vi "KE622x -- Delta Mode Get Params.vi"(0 "Resource In":refnum<visa-resource-name>, 1 "Check For SCPI Errors? (T)":bool=TRUE, 11 "error in (no error)":errorcluster) -> (4 "Resource Out (dupl)":refnum<visa-resource-name>, 8 "Delta Mode Params":T1={"High Level (A)"=0.001, "Low Level (A)"=-0.001, "Delay (s)"=0.002, "Num Cycles Mode"=enum."Finite Count", "Finite Count"=1, "Abort On\nCompliance?"=FALSE, "Cold Swithing\nMode Enabled?"=FALSE} {"Finite Count" min=1 max=65536; "Low Level (A)" min=-0.105 max=0.0 format="%.3p"; "High Level (A)" min=0.0 max=0.105 format="%.3p"; "Delay (s)" min=0.001 max=9999.999 format="%.3f"}, 15 "error out":errorcluster)   [LabVIEW 2020, in "Keithley 622x.lvlib"]
doc: "Returns the parameters for 'Delta' measurements. Note that performing this measurement implies that the 622x is being used in conjuction with a 2182/2182A nano-voltmeter."
uses:
  Keithley 622x.lvlib
  Typedefs/KE622x -- Delta Mode Params.ctl
  Low Level/Typedefs/KE622x -- Delta PDelta Mode High Level.ctl
  Low Level/Typedefs/KE622x -- Delta PDelta Mode Low Level.ctl
  Low Level/Typedefs/KE622x -- Delta DCon Mode Delay.ctl
  Low Level/Typedefs/KE622x -- Delta PDelta Mode Num Cycles Mode.ctl
  Low Level/Typedefs/KE622x -- Delta PDelta Mode Num Cycles.ctl
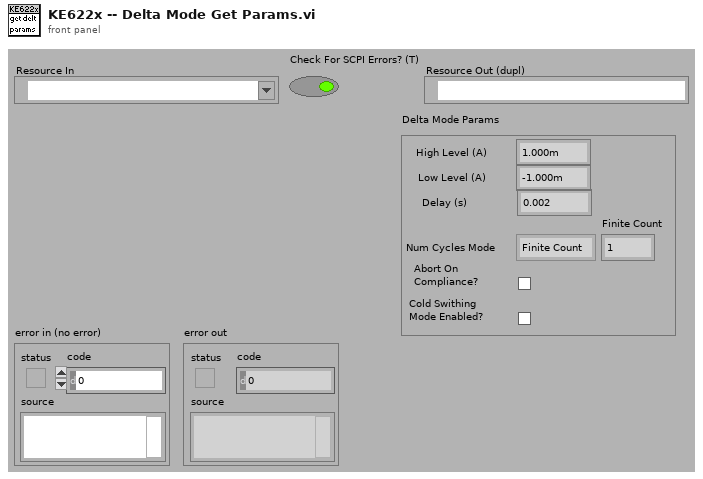
[diagram p1: front panel]
types:
  T1 = typedef "Keithley 622x.lvlib/KE622x -- Delta Mode Params.ctl" = cluster{"High Level (A)":T2, "Low Level (A)":T3, "Delay (s)":T4, "Num Cycles Mode":T5, "Finite Count":T6, "Abort On\nCompliance?":bool, "Cold Swithing\nMode Enabled?":bool}
  T2 = typedef "Keithley 622x.lvlib/KE622x -- Delta PDelta Mode High Level.ctl" = dbl
  T3 = typedef "Keithley 622x.lvlib/KE622x -- Delta PDelta Mode Low Level.ctl" = dbl
  T4 = typedef "Keithley 622x.lvlib/KE622x -- Delta DCon Mode Delay.ctl" = dbl
  T5 = typedef "Keithley 622x.lvlib/KE622x -- Delta PDelta Mode Num Cycles Mode.ctl" = enum16{"Finite Count", "Infinite"}
  T6 = typedef "Keithley 622x.lvlib/KE622x -- Delta PDelta Mode Num Cycles.ctl" = u32
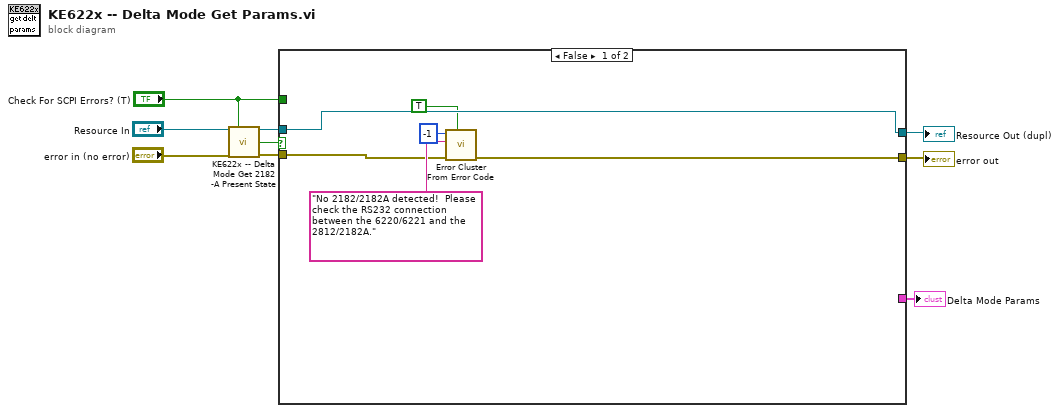
[diagram p0: block diagram]
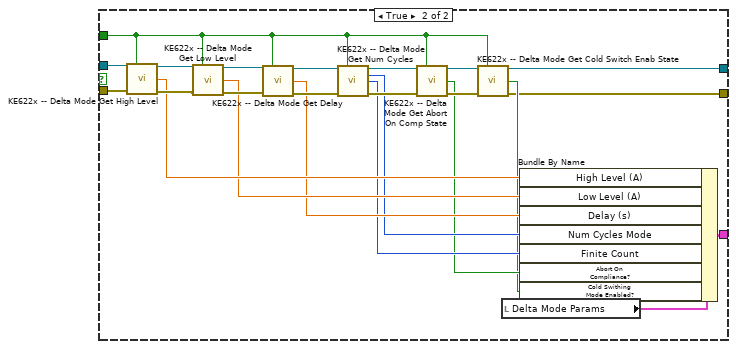
[diagram p2: hidden frame]
diagram:
  n1 = call "KE622x -- Delta Mode Get 2182 -A Present State.vi"("Resource In"="Resource In", "Check For SCPI Errors? (T)"="Check For SCPI Errors? (T)", "error in (no error)"="error in (no error)") -> ("Resource Out (dupl)"=w6:refnum<visa-resource-name>, "2182/2182A Present?"=w3:bool, "error out"=w5:errorcluster)  [unwired: 10 in]
  n2 = case shown="False" w3 {
    tunnel: [_ w21] -> w9
    tunnel: w6 -> [w11 w20]
    tunnel: w5 -> [w14 w19]
    tunnel: "Check For SCPI Errors? (T)" -> [_ w18]
    tunnel: [w12 w16] -> w2
    tunnel: [w11 w17] -> w1
    frame False {
      n3 = call <vilib>:"Error Cluster From Error Code.vi"("show call chain? (False)"=TRUE, "error in (no error)"=w14, "error message (\"\")"="No 2182/2182A detected!  Please check the RS232 connection between the 6220/6221 and the 2812/2182A.", "error code (0)"=-1) -> ("error out"=w12:errorcluster)  [unwired: 5 in]
    }
    frame True {
      n4 = call "KE622x -- Delta Mode Get High Level.vi"("Resource In"=w20, "Check For SCPI Errors? (T)"=w18, "error in (no error)"=w19) -> ("Resource Out (dupl)"=w39:refnum<visa-resource-name>, "High Level (A)"=w28:T2, "error out"=w38:errorcluster)  [unwired: 10 in]
      n5 = call "KE622x -- Delta Mode Get Low Level.vi"("Resource In"=w39, "Check For SCPI Errors? (T)"=w18, "error in (no error)"=w38) -> ("Resource Out (dupl)"=w37:refnum<visa-resource-name>, "Low Level (A)"=w27:T3, "error out"=w36:errorcluster)  [unwired: 10 in]
      n6 = call "KE622x -- Delta Mode Get Delay.vi"("Resource In"=w37, "Check For SCPI Errors? (T)"=w18, "error in (no error)"=w36) -> ("Resource Out (dupl)"=w35:refnum<visa-resource-name>, "Delay (s)"=w26:T4, "error out"=w34:errorcluster)  [unwired: 10 in]
      n7 = call "KE622x -- Delta Mode Get Num Cycles.vi"("Resource In"=w35, "Check For SCPI Errors? (T)"=w18, "error in (no error)"=w34) -> ("Resource Out (dupl)"=w31:refnum<visa-resource-name>, "Num Cycles Mode"=w25:T5, "Finite Count"=w24:T6, "error out"=w30:errorcluster)  [unwired: 9 in]
      n8 = call "KE622x -- Delta Mode Get Abort On Comp State.vi"("Resource In"=w31, "Check For SCPI Errors? (T)"=w18, "error in (no error)"=w30) -> ("Resource Out (dupl)"=w33:refnum<visa-resource-name>, "Abort On Compliance?"=w23:bool, "error out"=w32:errorcluster)  [unwired: 10 in]
      n9 = call "KE622x -- Delta Mode Get Cold Switch Enab State.vi"("Resource In"=w33, "Check For SCPI Errors? (T)"=w18, "error in (no error)"=w32) -> ("Resource Out (dupl)"=w17:refnum<visa-resource-name>, "Cold Switching Mode Enabled?"=w22:bool, "error out"=w16:errorcluster)  [unwired: 10 in]
      n10 = local read "Delta Mode Params"() -> (w29:T1)
      n11 = Bundle By Name(cluster=w29, "High Level (A)"=w28, "Low Level (A)"=w27, "Delay (s)"=w26, "Num Cycles Mode"=w25, "Finite Count"=w24, "Abort On\nCompliance?"=w23, "Cold Swithing\nMode Enabled?"=w22) -> (w21:T1)
    }
  }
  "Delta Mode Params" <- w9
  "Resource Out (dupl)" <- w1
  "error out" <- w2
